vi "Curs. and anott. vis. (FGV).vi"(8 "error in (no error)":errorcluster, 10 "Enum":T2(ring), 11 "cursors visibility in":T1) -> (0 "error out":errorcluster, 2 "anott. visibility array out":bool[](array[boolean]), 3 "cursors visibility out":T1)   [LabVIEW 2014]
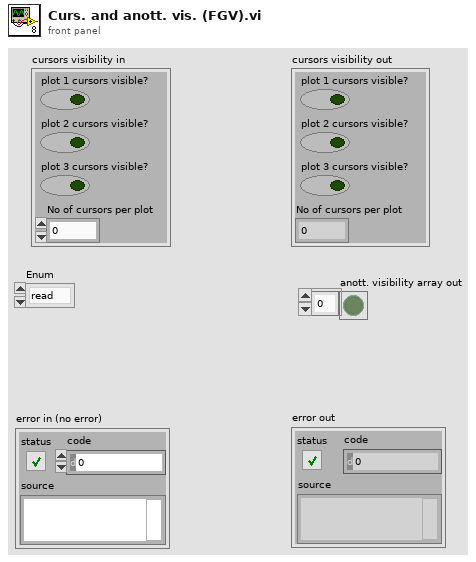
[diagram p1: front panel]
types:
  T1 = cluster{"plot 1 cursors visible? ":bool, "plot 2 cursors visible?":bool, "plot 3 cursors visible?":bool, "No of cursors per plot":i32}
  T2 = enum16{"read", "write", "write number of cursors per plot only"}
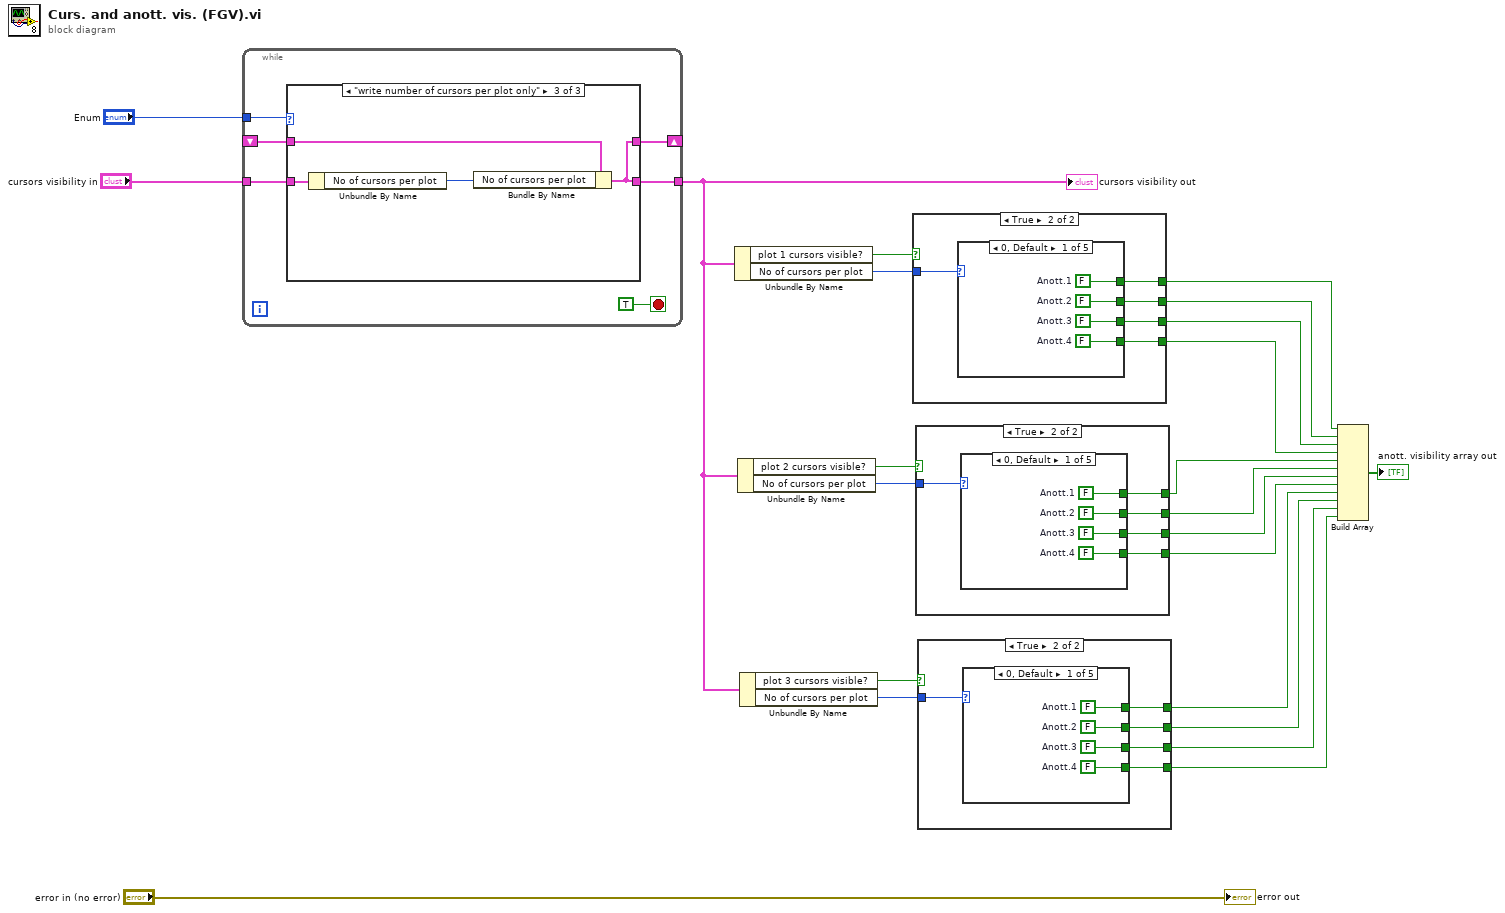
[diagram p0: block diagram]
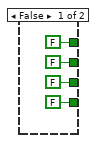
[diagram p2: hidden frame]
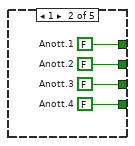
[diagram p3: hidden frame]
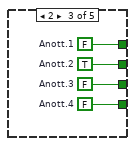
[diagram p4: hidden frame]
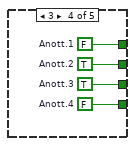
[diagram p5: hidden frame]
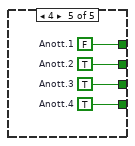
[diagram p6: hidden frame]
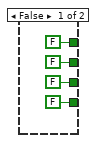
[diagram p7: hidden frame]
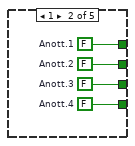
[diagram p8: hidden frame]
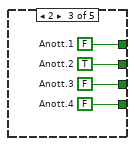
[diagram p9: hidden frame]
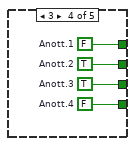
[diagram p10: hidden frame]
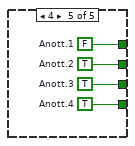
[diagram p11: hidden frame]
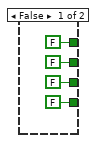
[diagram p12: hidden frame]
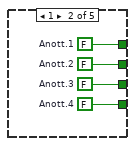
[diagram p13: hidden frame]
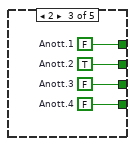
[diagram p14: hidden frame]
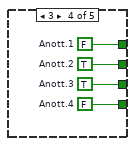
[diagram p15: hidden frame]
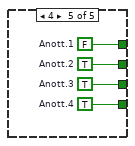
[diagram p16: hidden frame]
diagram:
  n1 = while {
    tunnel: "Enum" -> [w28]
    tunnel: "cursors visibility in" -> [w26]
    shift-right: [w27] -> _
    shift-left: _ -> [w25]
    tunnel: [w24] -> w14
    stop <- TRUE stop-if-true
    n2 = case shown="\"write number of cursors per plot only\"" w28 {
      tunnel: [w30 w31 w33] -> w27
      tunnel: w26 -> [_ w31 w34]
      tunnel: w25 -> [w30 _ w35]
      tunnel: [w30 w31 w33] -> w24
      frame "read", Default {
      }
      frame "write" {
      }
      frame "write number of cursors per plot only" {
        n3 = Unbundle By Name(w34) -> ("No of cursors per plot"=w32:i32)
        n4 = Bundle By Name(cluster=w35, "No of cursors per plot"=w32) -> (w33:T1)
      }
    }
  }
  "cursors visibility out" <- w14
  n5 = Unbundle By Name(w14) -> ("plot 1 cursors visible?"=w20:bool, "No of cursors per plot"=w19:i32)
  n6 = Unbundle By Name(w14) -> ("plot 2 cursors visible?"=w17:bool, "No of cursors per plot"=w18:i32)
  n7 = Unbundle By Name(w14) -> ("plot 3 cursors visible?"=w16:bool, "No of cursors per plot"=w15:i32)
  n8 = case shown="True" w20 {
    tunnel: w19 -> [_ w44]
    tunnel: [FALSE ("Anott.1") w43] -> w13
    tunnel: [FALSE ("Anott.2") w42] -> w12
    tunnel: [FALSE ("Anott.3") w41] -> w11
    tunnel: [FALSE ("Anott.4") w40] -> w10
    frame False {
    }
    frame True {
      n9 = case shown="0, Default" w44 {
        tunnel: [w48 w52 w56 w60 w61] -> w43
        tunnel: [w47 w51 w55 w59 w62] -> w42
        tunnel: [w46 w50 w54 w58 w63] -> w41
        tunnel: [w45 w49 w53 w57 w64] -> w40
        frame 0, Default {
          w45 = FALSE  # Anott.4
          w46 = FALSE  # Anott.3
          w47 = FALSE  # Anott.2
          w48 = FALSE  # Anott.1
        }
        frame 1 {
          w49 = FALSE  # Anott.4
          w50 = FALSE  # Anott.3
          w51 = FALSE  # Anott.2
          w52 = FALSE  # Anott.1
        }
        frame 2 {
          w53 = FALSE  # Anott.4
          w54 = FALSE  # Anott.3
          w55 = TRUE  # Anott.2
          w56 = FALSE  # Anott.1
        }
        frame 3 {
          w57 = FALSE  # Anott.4
          w58 = TRUE  # Anott.3
          w59 = TRUE  # Anott.2
          w60 = FALSE  # Anott.1
        }
        frame 4 {
          w64 = TRUE  # Anott.4
          w63 = TRUE  # Anott.3
          w62 = TRUE  # Anott.2
          w61 = FALSE  # Anott.1
        }
      }
    }
  }
  n10 = case shown="True" w17 {
    tunnel: w18 -> [_ w73]
    tunnel: [FALSE ("Anott.1") w72] -> w9
    tunnel: [FALSE ("Anott.2") w71] -> w8
    tunnel: [FALSE ("Anott.3") w70] -> w7
    tunnel: [FALSE ("Anott.4") w69] -> w6
    frame False {
    }
    frame True {
      n11 = case shown="0, Default" w73 {
        tunnel: [w77 w81 w85 w89 w90] -> w72
        tunnel: [w76 w80 w84 w88 w91] -> w71
        tunnel: [w75 w79 w83 w87 w92] -> w70
        tunnel: [w74 w78 w82 w86 w93] -> w69
        frame 0, Default {
          w74 = FALSE  # Anott.4
          w75 = FALSE  # Anott.3
          w76 = FALSE  # Anott.2
          w77 = FALSE  # Anott.1
        }
        frame 1 {
          w78 = FALSE  # Anott.4
          w79 = FALSE  # Anott.3
          w80 = FALSE  # Anott.2
          w81 = FALSE  # Anott.1
        }
        frame 2 {
          w82 = FALSE  # Anott.4
          w83 = FALSE  # Anott.3
          w84 = TRUE  # Anott.2
          w85 = FALSE  # Anott.1
        }
        frame 3 {
          w86 = FALSE  # Anott.4
          w87 = TRUE  # Anott.3
          w88 = TRUE  # Anott.2
          w89 = FALSE  # Anott.1
        }
        frame 4 {
          w93 = TRUE  # Anott.4
          w92 = TRUE  # Anott.3
          w91 = TRUE  # Anott.2
          w90 = FALSE  # Anott.1
        }
      }
    }
  }
  n12 = case shown="True" w16 {
    tunnel: w15 -> [_ w102]
    tunnel: [FALSE ("Anott.1") w101] -> w5
    tunnel: [FALSE ("Anott.2") w100] -> w4
    tunnel: [FALSE ("Anott.3") w99] -> w3
    tunnel: [FALSE ("Anott.4") w98] -> w2
    frame False {
    }
    frame True {
      n13 = case shown="0, Default" w102 {
        tunnel: [w106 w110 w114 w118 w119] -> w101
        tunnel: [w105 w109 w113 w117 w120] -> w100
        tunnel: [w104 w108 w112 w116 w121] -> w99
        tunnel: [w103 w107 w111 w115 w122] -> w98
        frame 0, Default {
          w103 = FALSE  # Anott.4
          w104 = FALSE  # Anott.3
          w105 = FALSE  # Anott.2
          w106 = FALSE  # Anott.1
        }
        frame 1 {
          w107 = FALSE  # Anott.4
          w108 = FALSE  # Anott.3
          w109 = FALSE  # Anott.2
          w110 = FALSE  # Anott.1
        }
        frame 2 {
          w111 = FALSE  # Anott.4
          w112 = FALSE  # Anott.3
          w113 = TRUE  # Anott.2
          w114 = FALSE  # Anott.1
        }
        frame 3 {
          w115 = FALSE  # Anott.4
          w116 = TRUE  # Anott.3
          w117 = TRUE  # Anott.2
          w118 = FALSE  # Anott.1
        }
        frame 4 {
          w122 = TRUE  # Anott.4
          w121 = TRUE  # Anott.3
          w120 = TRUE  # Anott.2
          w119 = FALSE  # Anott.1
        }
      }
    }
  }
  n14 = Build Array(w13, w12, w11, w10, w9, w8, w7, w6, w5, w4, w3, w2) -> (→"anott. visibility array out":bool[])
  "error out" <- "error in (no error)"
